vi "basic.vi"() -> ()   [LabVIEW 2019]
panel:
  out "number(0-100)":dbl
  out "number(0-10_":dbl
  out "number(0-1)":dbl
  out "-X":dbl
  out "sqrt(X)":dbl
  out "X^2":dbl
  out "X+1":dbl
  in  "X":dbl
  out "C/D":dbl
  out "E*2":dbl
  in  "E":dbl
  out "C-D":dbl
  in  "D":dbl
  in  "C":dbl
  in  "B":dbl
  out "A+B":dbl
  in  "A":dbl
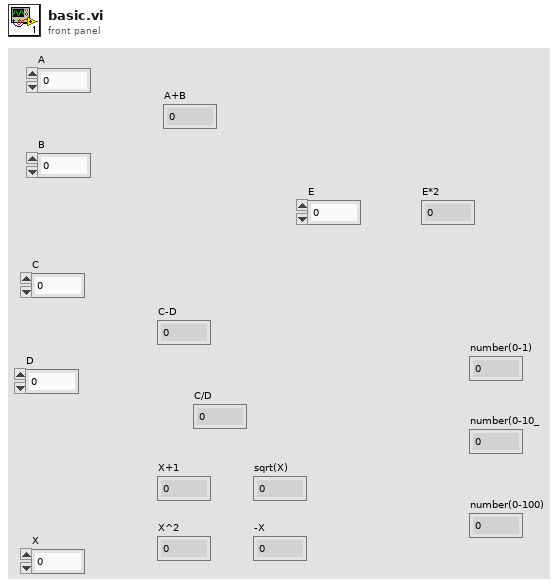
[diagram p1: front panel]
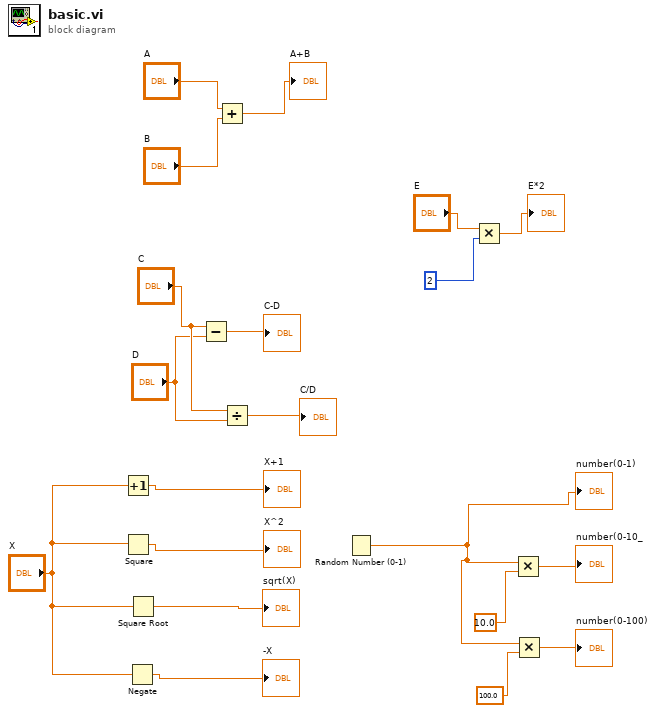
[diagram p0: block diagram]
diagram:
  n1 = Increment(x="X") -> (x+1=→"X+1":dbl)
  n2 = Square(x="X") -> (x^2=→"X^2":dbl)
  n3 = Negate(x="X") -> (-x=→"-X":dbl)
  n4 = Square Root(x="X") -> (sqrt(x)=→"sqrt(X)":dbl)
  n5 = Subtract(x="C", y="D") -> (x-y=→"C-D":dbl)
  n6 = Add(x="A", y="B") -> (x+y=→"A+B":dbl)
  n7 = Divide(x="C", y="D") -> (x/y=→"C/D":dbl)
  n8 = Random Number (0-1)() -> (number: 0 to 1=w3:dbl)
  "number(0-1)" <- w3
  n9 = Multiply(x="E", y=2) -> (x*y=→"E*2":dbl)
  n10 = Multiply(x=w3, y=10.0) -> (x*y=→"number(0-10_":dbl)
  n11 = Multiply(x=w3, y=100.0) -> (x*y=→"number(0-100)":dbl)
